vi "Set DefaultValue.vi"(8 "error in":errorcluster, 10 "Value":refnum<class "Value.lvclass">, 11 "Object Type in":refnum<class "ARRAY.lvclass">) -> (0 "error out":errorcluster, 3 "Object Type out":refnum<class "ARRAY.lvclass">)   [LabVIEW 2024, in "Electronic Datasheet.lvlib" / "ARRAY.lvclass"]
uses:
  ARRAY.lvclass
  Value/Value.lvclass
  Electronic Datasheet.lvlib
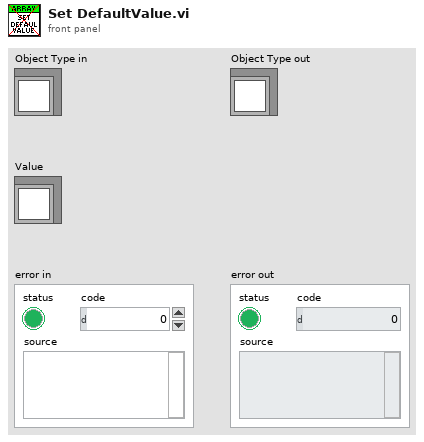
[diagram p1: front panel]
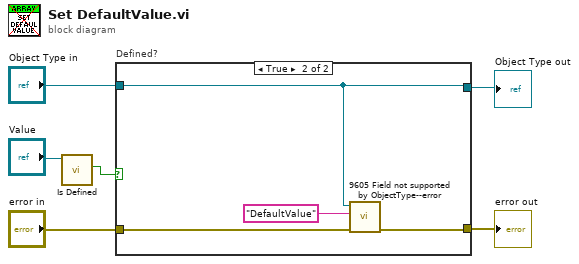
[diagram p0: block diagram]
diagram:
  n1 = call "Is Defined.vi"("Value in"="Value") -> ("Is Defined?"=w5:bool)  [unwired: 9 in, 1 out]
  n2 = case "Defined?" shown="True" w5 {
    tunnel: [w8 w11] -> w1
    tunnel: "Object Type in" -> [w7 w9]
    tunnel: [w7 w9] -> w2
    tunnel: "error in" -> [w8 w12]
    frame False {
    }
    frame True {
      n3 = call "9605 Field not supported by ObjectType--error.vi"("error in"=w12, "Field Name"="DefaultValue" ("Field name"), "Object Type Base"=w9) -> ("error out"=w11:errorcluster)  [unwired: 8 in]
    }
  }
  "Object Type out" <- w2
  "error out" <- w1
